vi "cDAQ_VI_Leo_Main.vi"() -> ()   [LabVIEW 2022 SP3]
uses:
  <vilib>/Analysis/baseanly.llb/Mean (DBL).vi
  <vilib>/DAQmx/read.llb/DAQmx Read (Analog 1D Wfm NChan NSamp).vi
  STOP_GLOBAL.vi
  <vilib>/addons/control/pid/pid.llb/PID Lead-Lag (DBL).vi
  <vilib>/addons/control/pid/pid.llb/PID (DBL).vi
  <vilib>/DAQmx/configure/timing.llb/DAQmx Timing (Sample Clock).vi
  <vilib>/DAQmx/miscellaneous.llb/DAQmx Fill In Error Info.vi
  <vilib>/Analysis/NI_AALBase.lvlib
  <vilib>/addons/control/pid/NI_PID_pid.lvlib
panel:
  out "Setpoint profile":dbl
  out "Voltage Output":dynamicdata(graph)
  out "Second Pressure Transducer":cluster{dbl[], dbl[]}(graph)
  out "Second Pressure Transducer":dynamicdata(graph)
  out "output":dbl format="%.2f"
  out "Servo Voltage Output":cluster{dbl[], dbl[]}(graph)
  out "Elapsed Time (s)":dbl
  in  "Tab Control":T1(tab)
  in  "Channel Array":dbl[](array[numeric]) format="%_3g"
  out "error out 5":errorcluster
  in  "stop":bool
  out "Output":dbl(slide) scale=0.0..5.067
  out "elapsed time (s)":dbl format="%.3f"
  in  "reinitialize? (F)":bool
  out "Waveform Chart 2":cluster{"setpoint":dbl, dbl}(graph) caption="Waveform Chart"
  out "Process Variable vs Setpoint":cluster{dbl[], dbl[]}[](graph)
  out "error out":errorcluster
  out "Steps on Needle 3":dbl[](array[numeric])
  in  "Error":dbl
  in  "Scaling Factor":dbl
  in  "x0":dbl
  out "element":dbl
  out "Process variable":dbl
  out "Setpoint":dbl
  in  "setpoint profile":cluster{"time (s)":dbl, "setpoint":dbl}[](array[cluster]) {"setpoint" format="%.2f"; "time (s)" format="%.3f"}
  in  "PID gains":T2={"proportional gain (Kc)"=1.0, "integral time (Ti, min)"=0.01, "derivative time (Td, min)"=0.0} {"derivative time (Td, min)" format="%.3f"; "integral time (Ti, min)" format="%.3f"; "proportional gain (Kc)" format="%.3f"}
  out "Steps on Servo":dbl[](array[numeric])
  out "Elapsed Time (s) 2":dbl caption="Elapsed Time (s)"
  out "HAS 3 SECONDS PASSED?":bool
  in  "PRESS TO START":bool
  out "All Channel Graph":cluster{dbl[], dbl[]}[](graph)
  out "Thrust":cluster{dbl[], dbl[]}(graph)
  out "Chamber Pressure":cluster{dbl[], dbl[]}(graph)
  out "Supply Pressure":cluster{dbl[], dbl[]}(graph)
  out "MassFlow":cluster{dbl[], dbl[]}(graph)
  out "Temperature":cluster{dbl[], dbl[]}(graph)
  out "error out 3":errorcluster caption="error out"
  out "error out 2":errorcluster
  in  "rate":dbl=1000.0 format="%0.2f"
  in  "number of samples":i32=100
  in  "File Format":string
  in  "File Name Out":string
  in  "Data Collection Folder":path
  out "Temperature":dynamicdata(graph)
  out "Numeric 2":i32
  out "Thrust lb":dynamicdata(graph)
  in  "Types of Testing":enum32{"Test Firing", "Cold Flow Rig"}(tab)
  out "Saving Data":bool
  out "Filename Out":path
  in  "Collect Data?":bool=TRUE caption="Enable"
  in  "Collect Data? 2":bool=TRUE caption="Enable"
  out "Saving Data":bool
  out "Filename Out":path
  out "Supply Pressure PSI":dynamicdata(graph)
  out "Mass Flow L/min":dynamicdata(graph)
  out "Chamber Pressure":dynamicdata(graph)
  # "Control Loop"
  # "DATA LOGGING INFORMATION"
  # "ANALOG VOLTAGE OUTPUT"
  # "RESULTS"
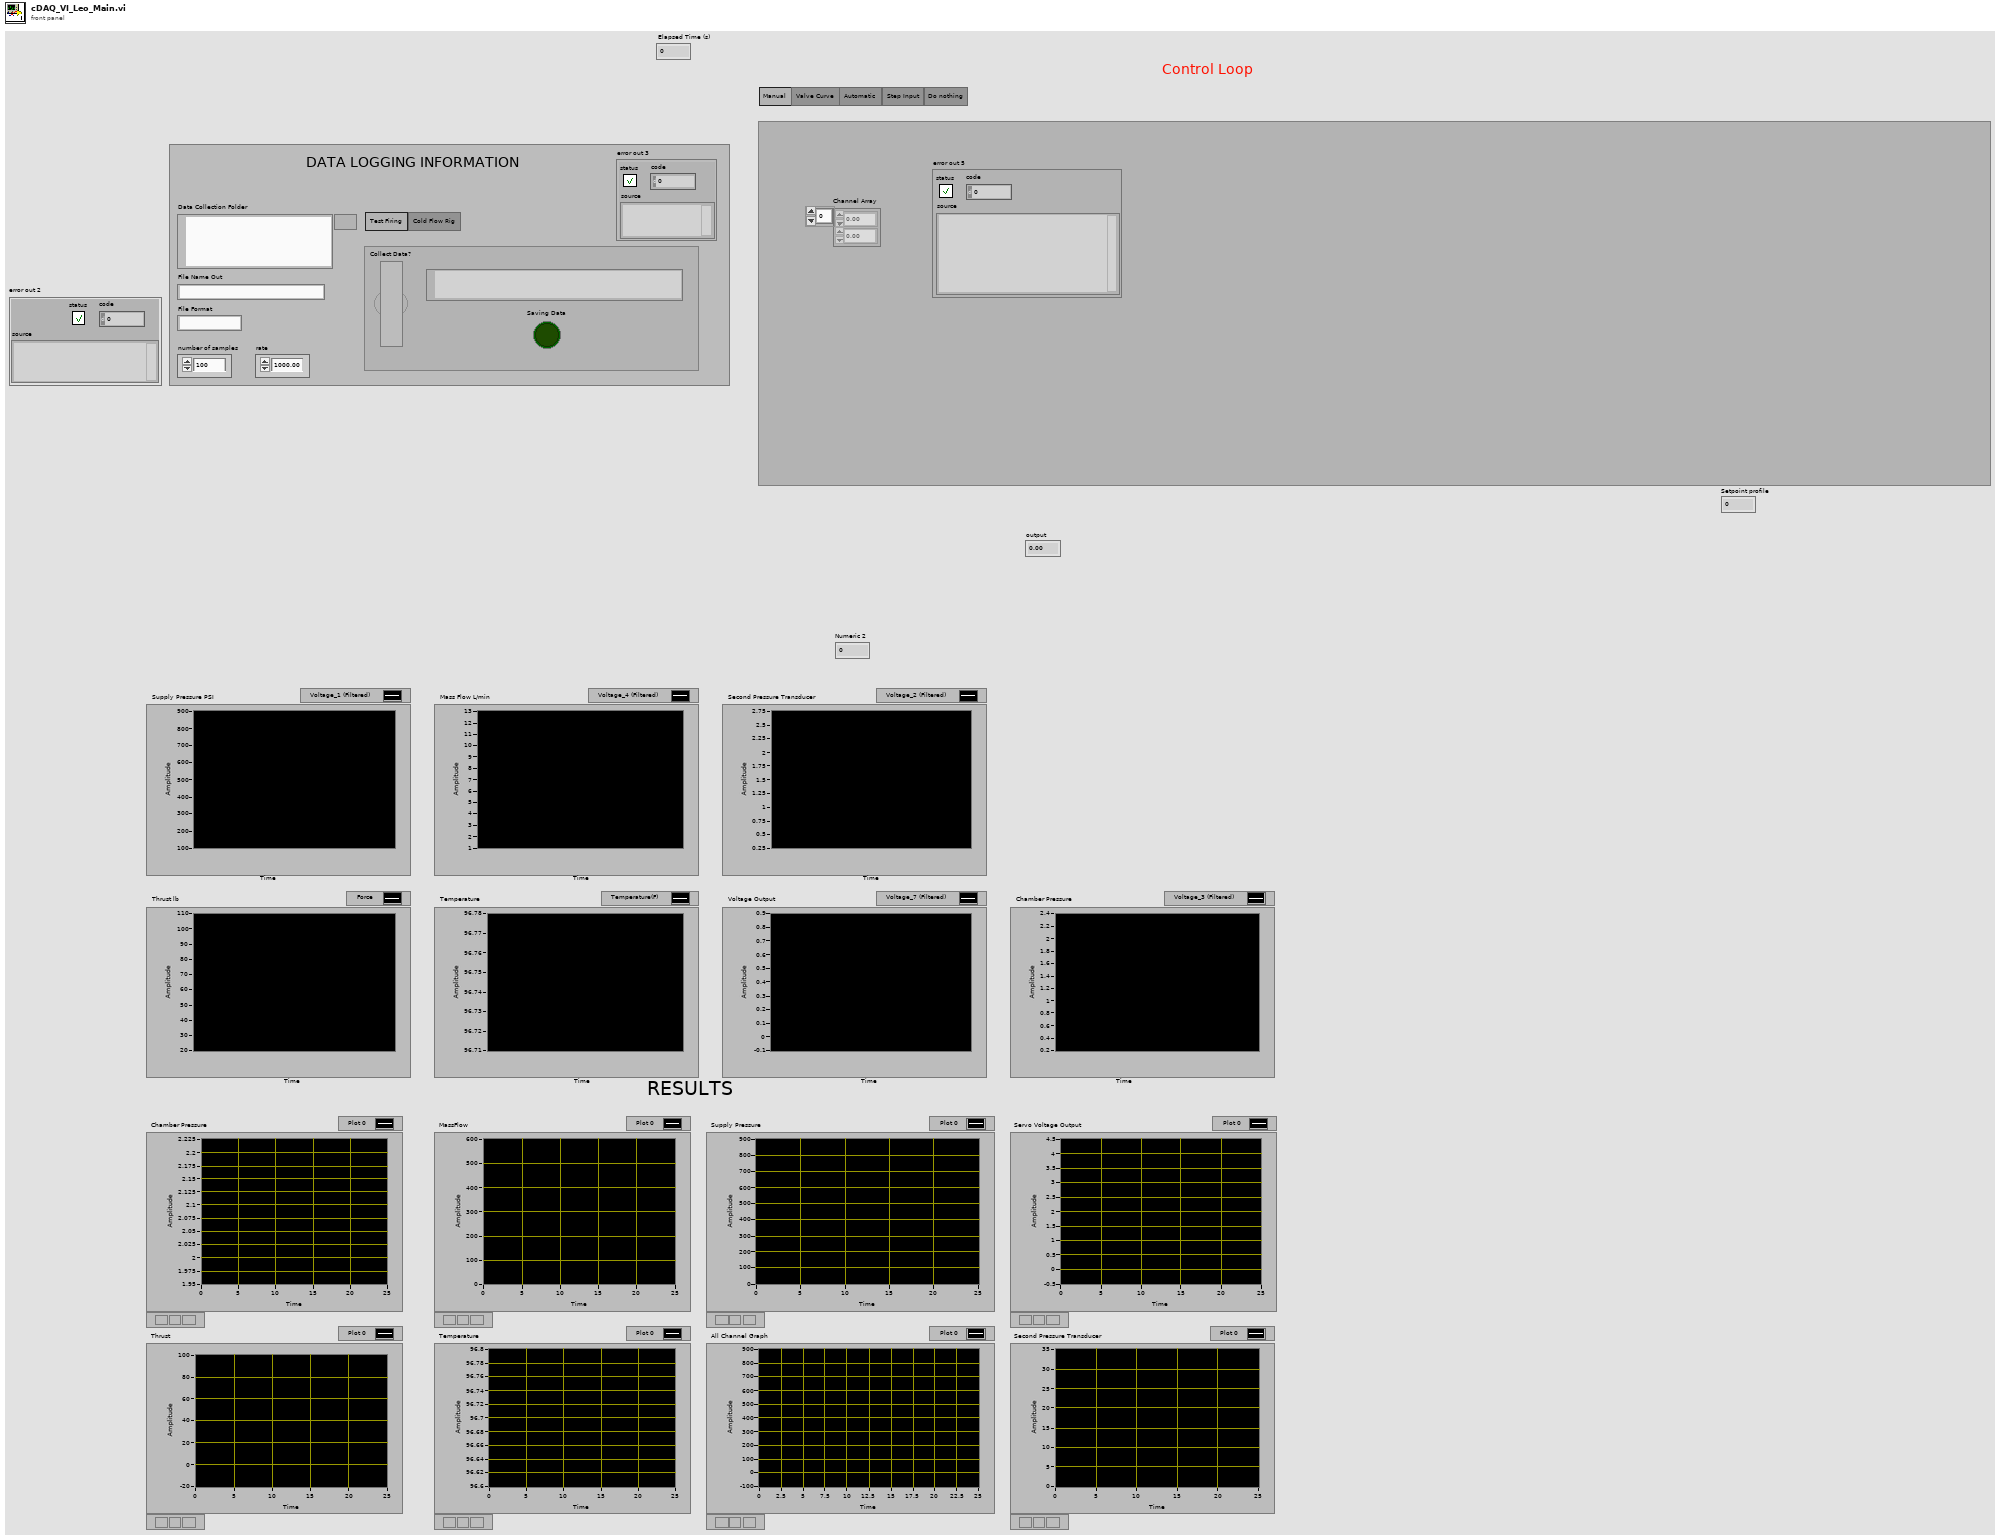
[diagram p1: front panel]
types:
  T1 = enum32{"Manual", "Valve Curve", "Automatic", "Step Input", "Do nothing"}
  T2 = cluster{"proportional gain (Kc)":dbl, "integral time (Ti, min)":dbl, "derivative time (Td, min)":dbl}
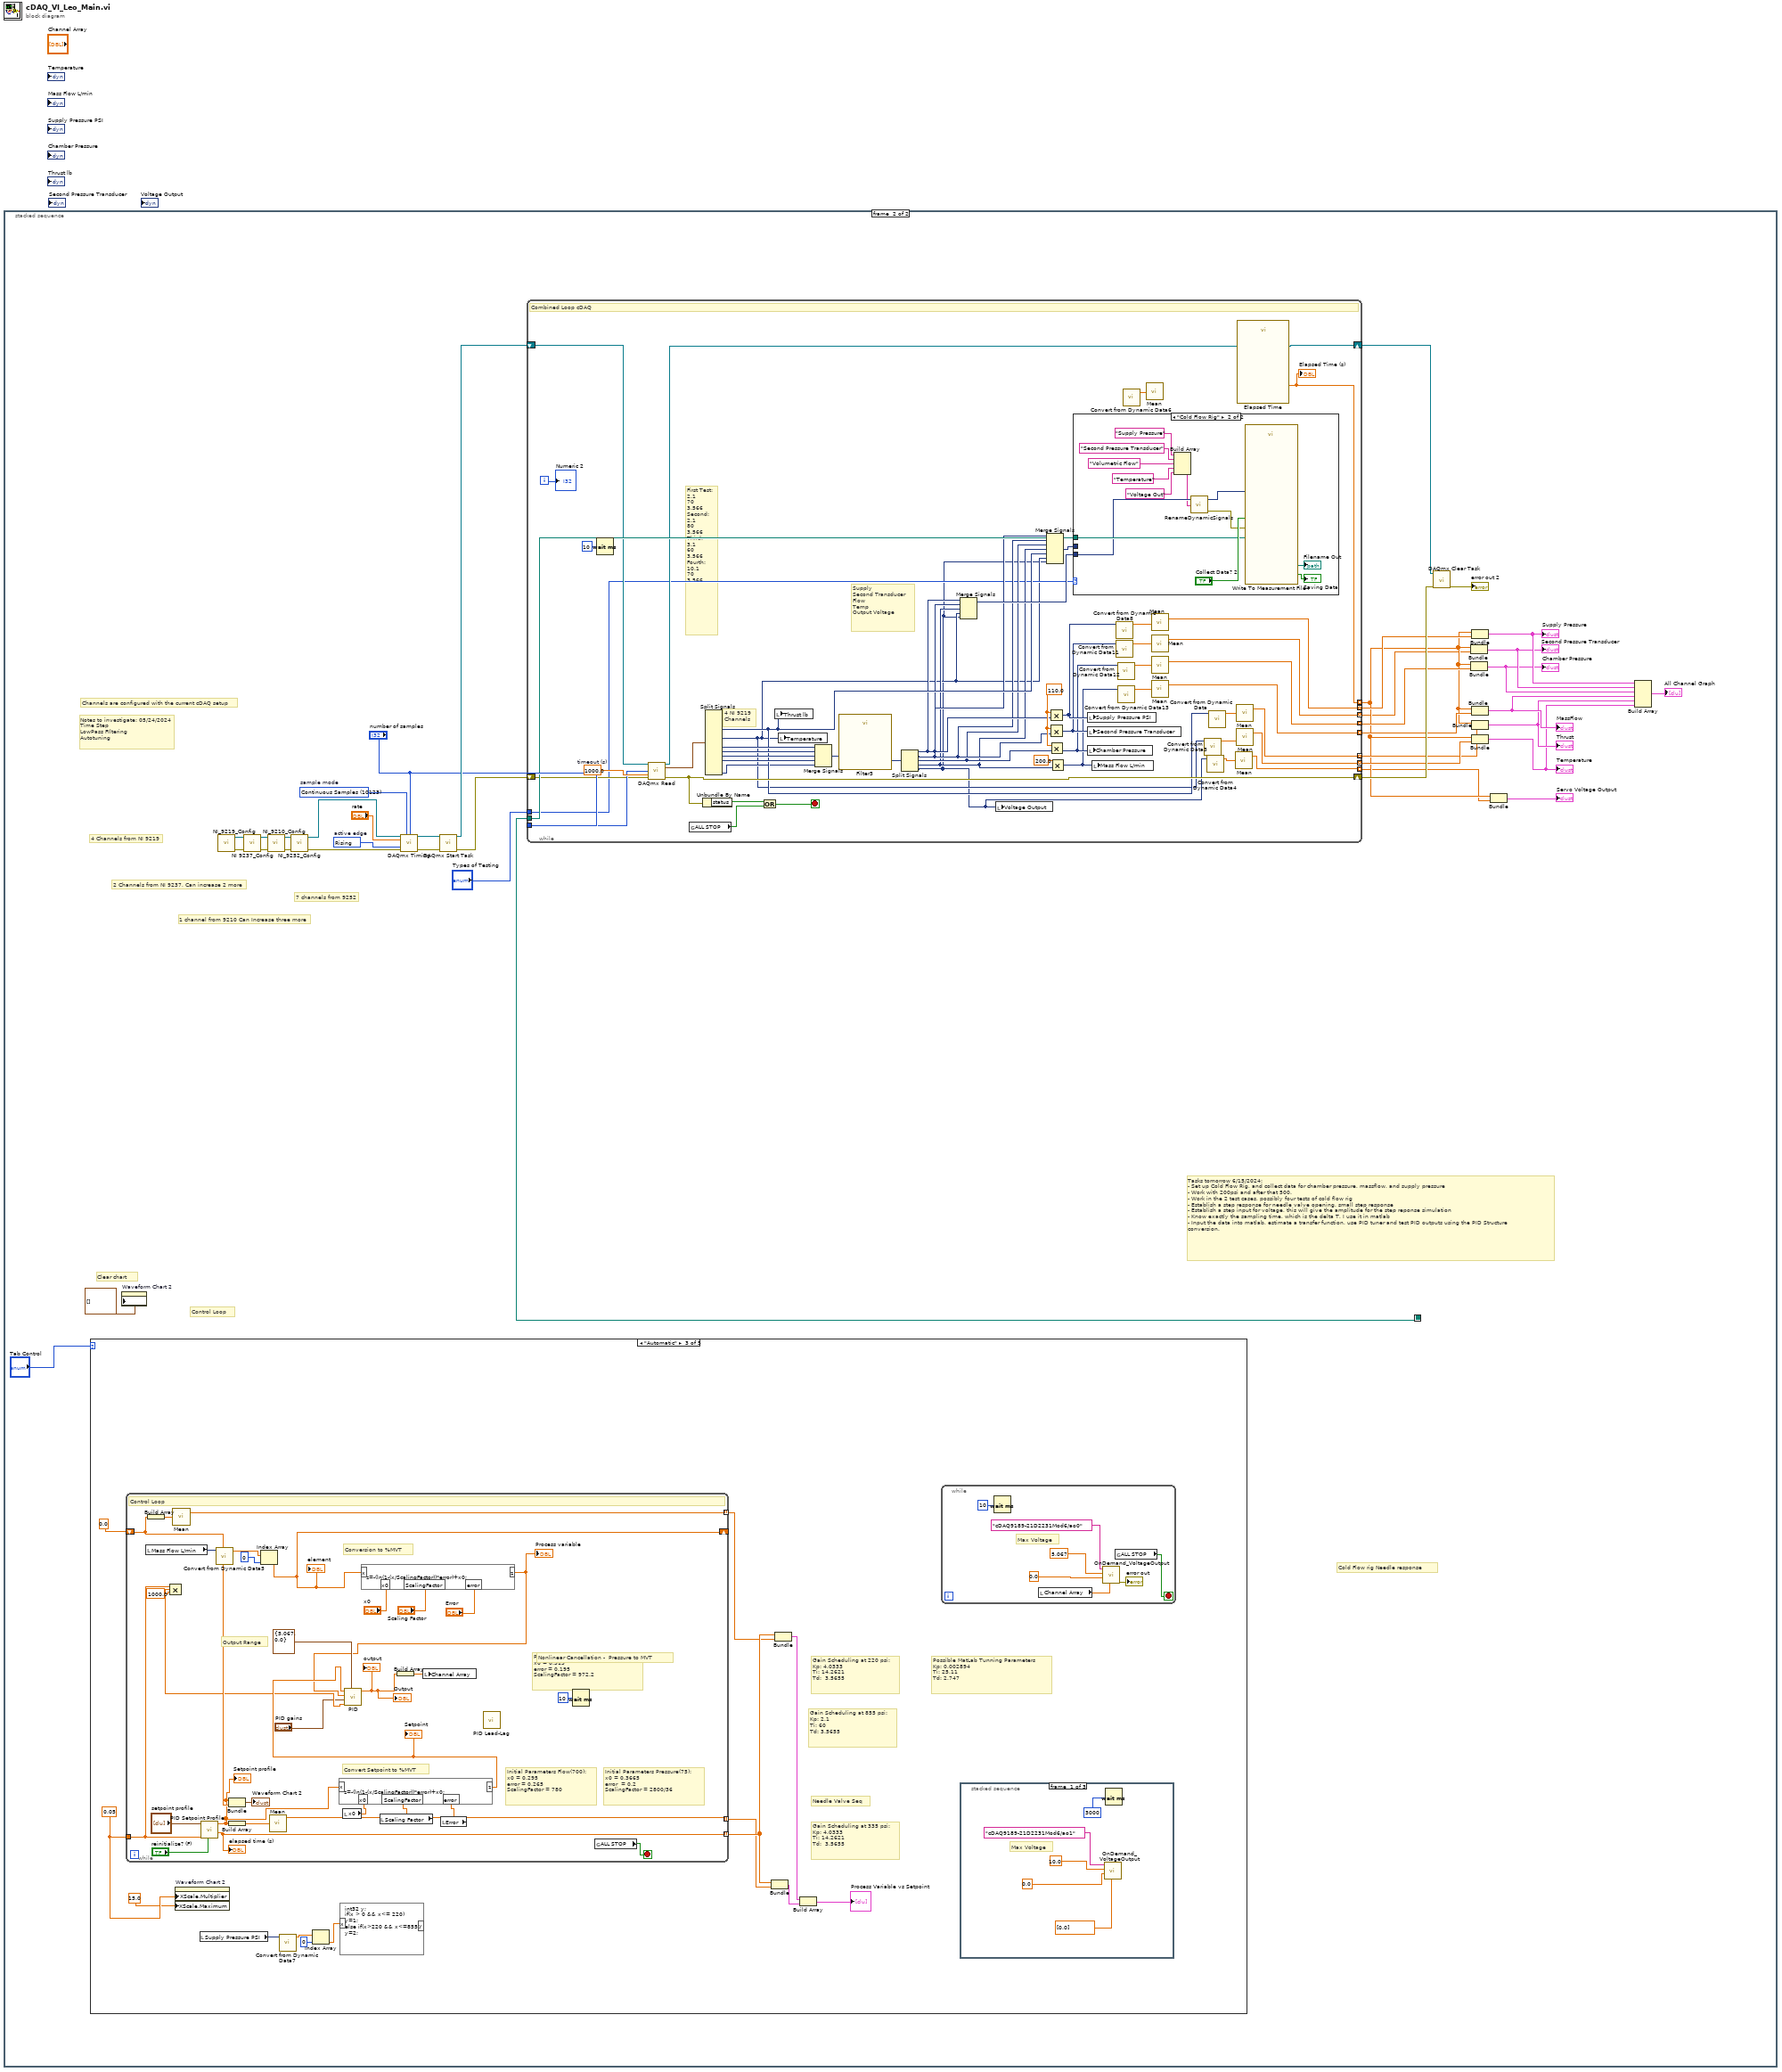
[diagram p0: block diagram]
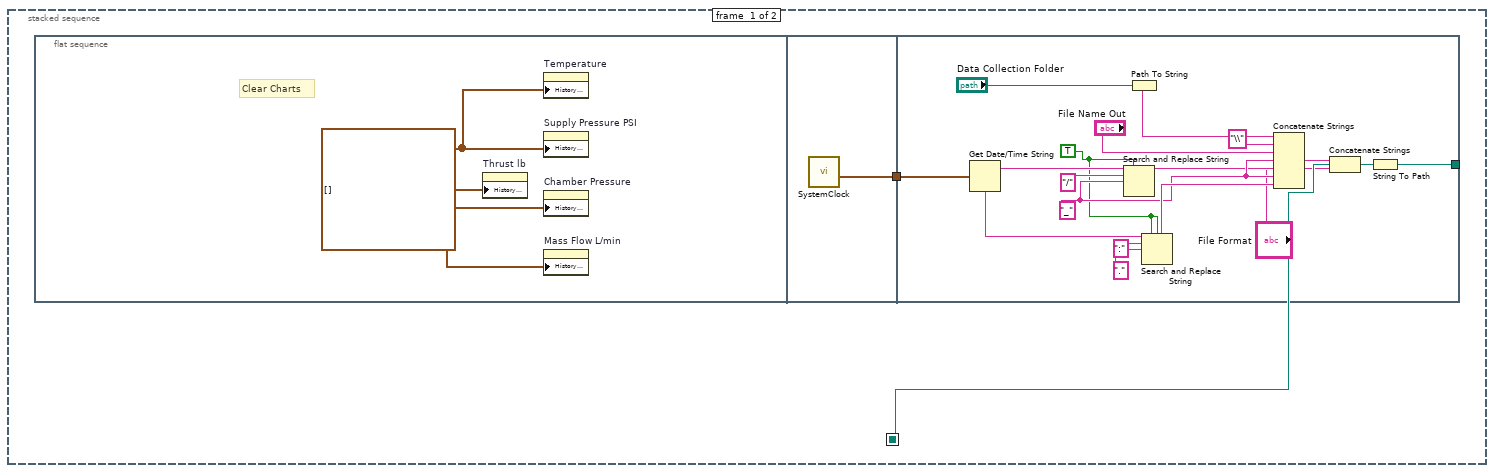
[diagram p2: hidden frame]
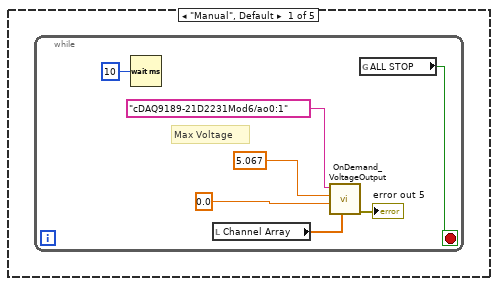
[diagram p3: hidden frame]
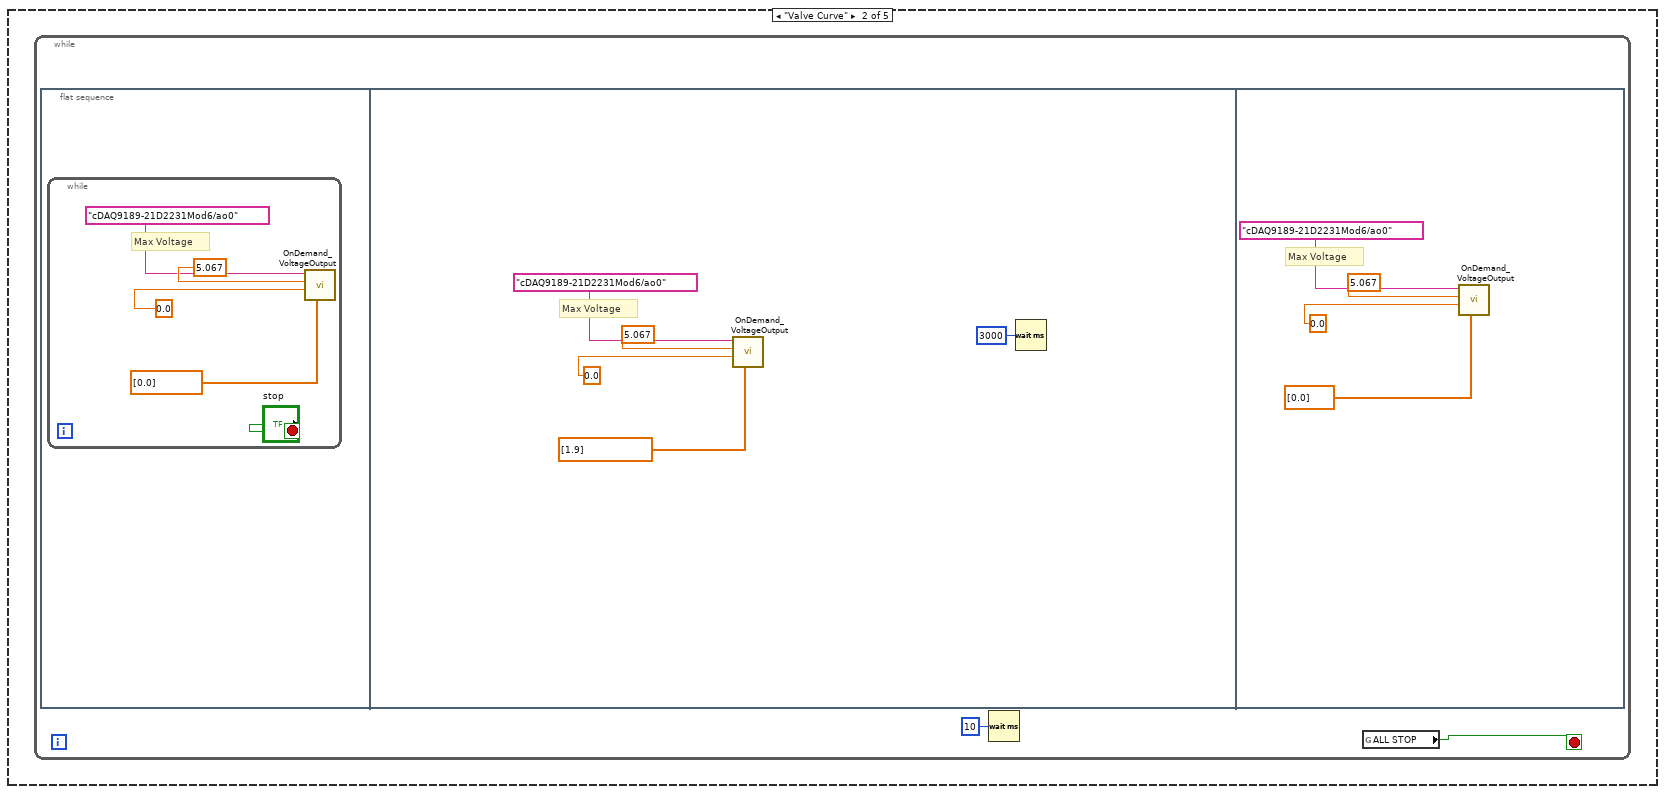
[diagram p4: hidden frame]
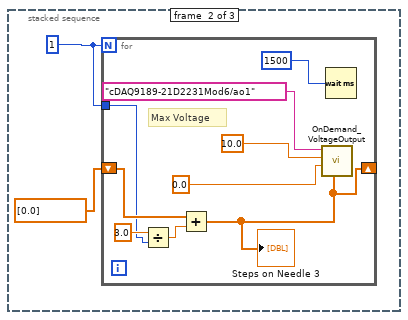
[diagram p5: hidden frame]
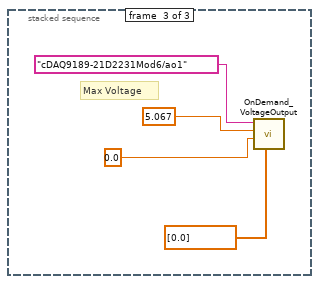
[diagram p6: hidden frame]
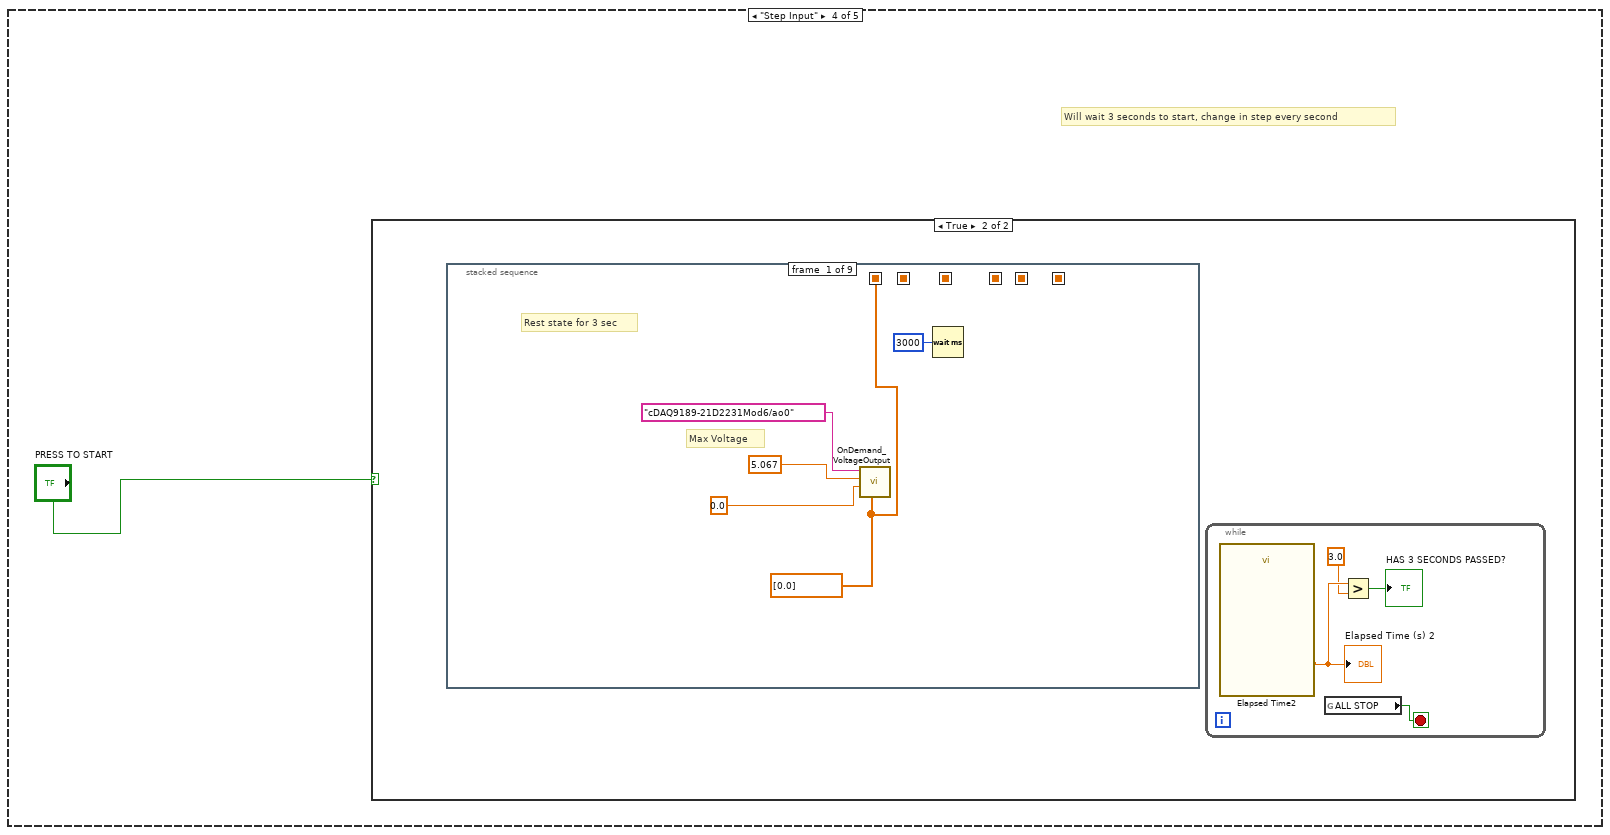
[diagram p7: hidden frame]
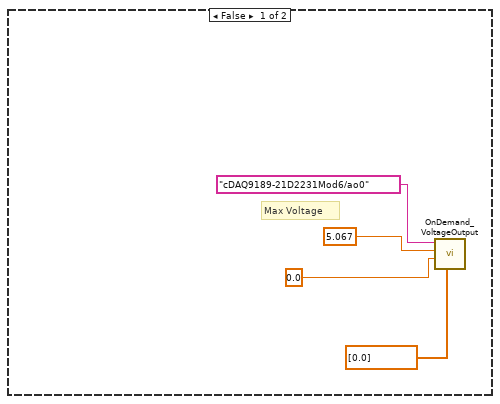
[diagram p8: hidden frame]
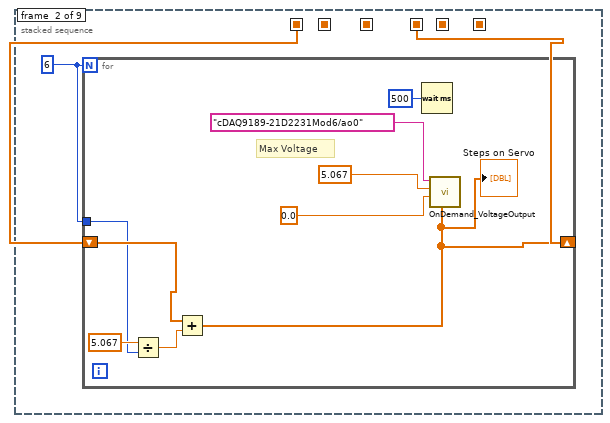
[diagram p9: hidden frame]
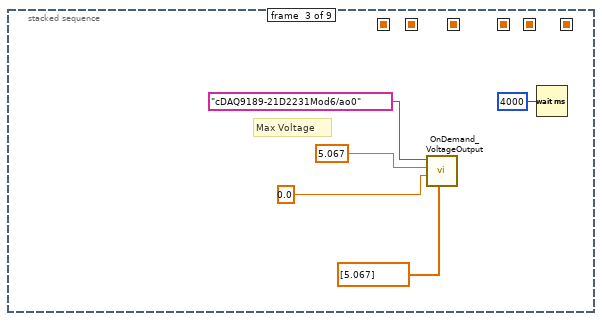
[diagram p10: hidden frame]
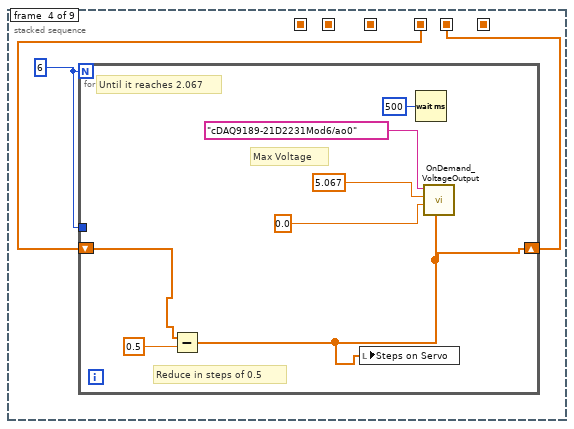
[diagram p11: hidden frame]
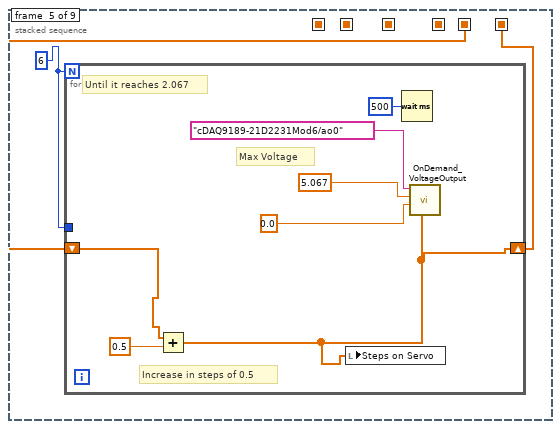
[diagram p12: hidden frame]
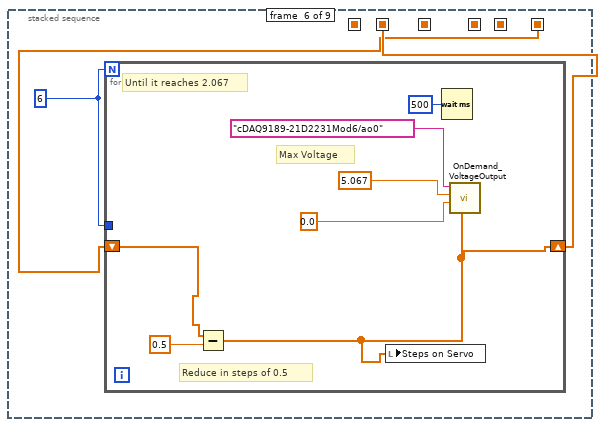
[diagram p13: hidden frame]
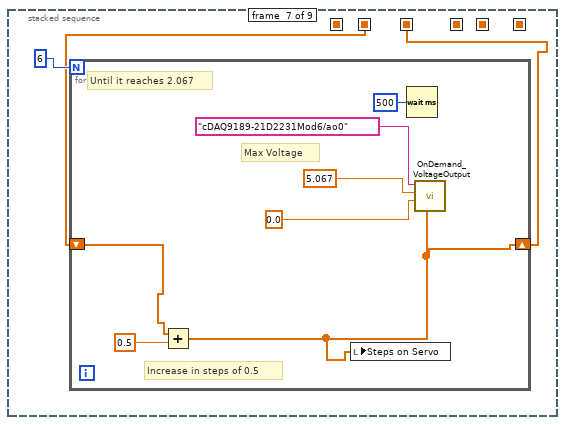
[diagram p14: hidden frame]
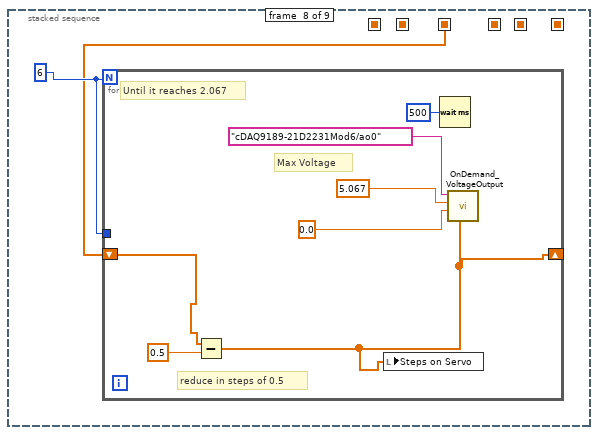
[diagram p15: hidden frame]
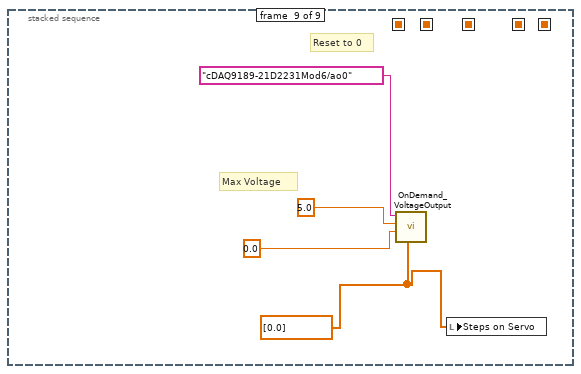
[diagram p16: hidden frame]
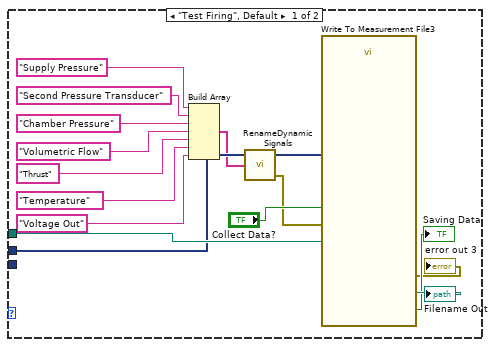
[diagram p18: hidden frame]
diagram:
  n1 = stacked-sequence {
    seq-local: [w1 _] -> [_ w60]
    frame #0 {
      n2 = flat-sequence {
        tunnel: [w4] -> w2
        tunnel: w2 -> [w11]
        tunnel: [w10] -> w1
        frame #0 {
          w3 = waveform(dbl)[] []
          # "Clear Charts"
          n3 = property on="Thrust lb" class="WFChart (strict)"("History Data"=w3) -> ()  [unwired: 2 in, 2 out]
          n4 = property on="Temperature" class="WFChart (strict)"("History Data"=w3) -> ()  [unwired: 2 in, 2 out]
          n5 = property on="Supply Pressure PSI" class="WFChart (strict)"("History Data"=w3) -> ()  [unwired: 2 in, 2 out]
          n6 = property on="Chamber Pressure" class="WFChart (strict)"("History Data"=w3) -> ()  [unwired: 2 in, 2 out]
          n7 = property on="Mass Flow L/min" class="WFChart (strict)"("History Data"=w3) -> ()  [unwired: 2 in, 2 out]
        }
        frame #1 {
          n8 = call "SystemClock.vi"() -> ("LabVIEW Time Stamp"=w4:timestamp)  [unwired: 9 in, 2 out]
        }
        frame #2 {
          w6 = TRUE ("replace all? (F)")
          w19 = "_" ("string")
          n9 = Get Date/Time String(seconds (now)=w11) -> (date string=w13:string, time string=w16:string)  [unwired: 2 in]
          n10 = Search and Replace String(replace all?=w6, input string=w13, search string="/", replace string=w19) -> (result string=w15:string)  [unwired: 4 in, 3 out]
          n11 = Path To String(path="Data Collection Folder") -> (string=w8:string)
          n12 = Search and Replace String(replace all?=w6, case sensitive?=w6, input string=w16, search string=":", replace string="." ("replace string (\"\")")) -> (result string=w20:string)  [unwired: 3 in, 3 out]
          n13 = Concatenate Strings(w8, "\\" ("string"), "File Name Out", w19, w15, w19, w20) -> (w21:string)
          n14 = Concatenate Strings(w21, "File Format") -> (w22:string)
          n15 = String To Path(string=w22) -> (path=w10:path)
        }
      }
    }
    frame #1 {
      w58 = 10123 items=["Finite Samples"=10178, "Continuous Samples"=10123, "Hardware Timed Single Point"=12522]  # sample mode
      w59 = 10280 items=["Rising"=10280, "Falling"=10171]  # active edge
      # "Cold Flow rig Needle response"
      # "Tasks tomorrow 6/15/2024:\n- Set up Cold Flow Rig, and collect data for chamber pressure, massflow, and supply pressure\n- Work with 200psi and after that 500.\n- Work in the 2 test cases, possibly four tests of cold flow rig\n- Establish a step response for needle valve opening, small step response\n- Establish a step input for voltage, this will give the amplitude for the step reponse simulation\n- Know exactly the sampling time, which is the delta T, I use it in matlab\n- Input the data into matlab, estimate a transfer function, use PID tuner and test PID outputs using the PID Structure\nconversion."
      # "Control Loop"
      # "Clear chart"
      # "Notes to investigate: 05/24/2024\nTime Step\nLowPass FIltering\nAutotuning"
      # "Channels are configured with the current cDAQ setup"
      # "7 channels from 9252"
      # "1 channel from 9210 Can Increase three more"
      # "2 Channels from NI 9237, Can increase 2 more"
      # "4 Channels from NI 9219"
      n16 = case shown="\"Automatic\"" "Tab Control" {
        frame "Manual", Default {
          n17 = while {
            stop <- w68 stop-if-true
            # "Max Voltage"
            n18 = Wait (ms)(milliseconds to wait=u32 10) -> ()  [unwired: 1 out]
            n19 = local read "Channel Array"() -> (w64:dbl[])
            n20 = call "OnDemand_VoltageOutput.vi"("Channel Array"=w64, "minimum voltage"=0.0, "maximum voltage"=5.067, "physical channels"="cDAQ9189-21D2231Mod6/ao0:1") -> ("error out"=→"error out 5":errorcluster)  [unwired: 7 in]
            n21 = global read "STOP_GLOBAL.vi" "ALL STOP"() -> (w68:bool)
          }
        }
        frame "Valve Curve" {
          n22 = while {
            stop <- w69 stop-if-true
            n23 = flat-sequence {
              frame #0 {
                n24 = while {
                  stop <- "stop" stop-if-true
                  # "Max Voltage"
                  n25 = call "OnDemand_VoltageOutput.vi"("Channel Array"=dbl[] [0.0], "minimum voltage"=0.0, "maximum voltage"=5.067, "physical channels"="cDAQ9189-21D2231Mod6/ao0") -> ()  [unwired: 7 in, 1 out]
                }
              }
              frame #1 {
                # "Max Voltage"
                n26 = call "OnDemand_VoltageOutput.vi"("Channel Array"=dbl[] [1.9], "minimum voltage"=0.0, "maximum voltage"=5.067, "physical channels"="cDAQ9189-21D2231Mod6/ao0") -> ()  [unwired: 7 in, 1 out]
                n27 = Wait (ms)(milliseconds to wait=u32 3000) -> ()  [unwired: 1 out]
              }
              frame #2 {
                # "Max Voltage"
                n28 = call "OnDemand_VoltageOutput.vi"("Channel Array"=dbl[] [0.0], "minimum voltage"=0.0, "maximum voltage"=5.067, "physical channels"="cDAQ9189-21D2231Mod6/ao0") -> ()  [unwired: 7 in, 1 out]
              }
            }
            n29 = Wait (ms)(milliseconds to wait=u32 10) -> ()  [unwired: 1 out]
            n30 = global read "STOP_GLOBAL.vi" "ALL STOP"() -> (w69:bool)
          }
        }
        frame "Automatic" {
          w97 = 0.05 ("dt (s)")
          # "Possible MatLab Tunning Parameters\nKp: 0.002894\nTi: 25.11\nTd: 2.747"
          # "Gain Scheduling at 335 psi:\nKp: 4.0333\nTi: 14.2621\nTd:  3.5655"
          # "Gain Scheduling at 855 psi:\nKp: 2.1\nTi: 60\nTd: 3.5655"
          # "Gain Scheduling at 220 psi:\nKp: 4.0333\nTi: 14.2621\nTd:  3.5655"
          # "Needle Valve Seq"
          n31 = while {
            shift-right: [w132] -> _
            shift-left: 0.0 -> [w149]
            tunnel: w97 -> [w152]
            tunnel: [w150] -> w93 mode=indexing
            tunnel: [w148] -> w91 mode=indexing
            tunnel: [w146] -> w92 mode=indexing
            stop <- w155 stop-if-true
            # "Possible parameters for 800 SLM:\nx0 = 0.315\nerror = 0.195\nScalingFactor = 972.2"
            # "Initial Parameters Pressure(75):\nx0 = 0.3665\nerror  = 0.2\nScalingFactor = 2800/36"
            # "Initial Parameters Flow(700):\nx0 = 0.295\nerror = 0.265\nScalingFactor = 780"
            # "Nonlinear Cancellation -  Pressure to MVT"
            # "Convert Setpoint to %MVT"
            # "Conversion to %MVT"
            # "Output Range"
            # "Control Loop"
            n32 = local read "Mass Flow L/min"() -> (w128:dynamicdata)
            n33 = Build Array(w149) -> (w147:dbl[])
            n34 = Multiply(x=w152, y=1000.0) -> (x*y=w136:dbl)
            n35 = call-poly <vilib>:"Mean.vi"("X"=w147) -> ("mean"=w148:dbl)  [unwired: 1 out]
            n36 = call <vilib>:"PID Setpoint Profile.vi"("reinitialize? (F)"="reinitialize? (F)", "dt (s)"=w152, "setpoint profile"="setpoint profile") -> ("elapsed time (s)"=w150:dbl, "setpoint"=w126:dbl)  [unwired: 3 in, 2 out]
            "elapsed time (s)" <- w150
            "Setpoint profile" <- w126
            n37 = call "Convert from Dynamic Data5"("Dynamic Data Type"=w128) -> ("Array"=w131:dbl[])  [unwired: 3 in]
            n38 = Bundle("setpoint"=w126, w149) -> (→"Waveform Chart 2":cluster{"setpoint":dbl, dbl})  [unwired: 1 in]
            n39 = Build Array(w126) -> (w143:dbl[])
            n40 = Index Array(array=w131, index=0) -> (element=w132:dbl)
            "element" <- w132
            n41 = call-poly <vilib>:"Mean.vi"("X"=w143) -> ("mean"=w146:dbl)  [unwired: 1 out]
            n42 = local read "x0"() -> (w142:dbl)
            n43 = formula code="z=-(ln(1-(x/ScalingFactor))*error)+x0;"("x"=w132, "x0"="x0", "ScalingFactor"="Scaling Factor", "error"="Error") -> ("z"=w129:dbl)
            "Process variable" <- w129
            n44 = local read "Scaling Factor"() -> (w141:dbl)
            n45 = local read "Error"() -> (w140:dbl)
            n46 = formula code="z=-(ln(1-(x/ScalingFactor))*error)+x0;"("x"=w126, "x0"=w142, "ScalingFactor"=w141, "error"=w140) -> ("z"=w137:dbl)
            "Setpoint" <- w137
            n47 = call-poly <vilib>:"PID.vi"("output range"=cluster{"output high":dbl, "output low":dbl} {"output high"=5.067, "output low"=0.0}, "dt (s)"=w136, "PID gains"="PID gains", "process variable"=w129, "setpoint"=w137) -> ("output"=w139:dbl)  [unwired: 5 in, 1 out]
            "Output" <- w139
            "output" <- w139
            n48 = Build Array(w139) -> (w151:dbl[])
            n49 = local write "Channel Array"(w151) -> ()
            n50 = call-poly <vilib>:"PID Lead-Lag.vi"() -> ()  [unwired: 8 in, 2 out]
            n51 = Wait (ms)(milliseconds to wait=u32 10) -> ()  [unwired: 1 out]
            n52 = global read "STOP_GLOBAL.vi" "ALL STOP"() -> (w155:bool)
          }
          n53 = property on="Waveform Chart 2" class="WFChart (strict)"("XScale.Multiplier"=w97, "XScale.Maximum"=15.0 ("X Scale.Range:Maximum")) -> ()  [unwired: 2 in, 2 out]
          n54 = local read "Supply Pressure PSI"() -> (w88:dynamicdata)
          n55 = call "Convert from Dynamic Data7"("Dynamic Data Type"=w88) -> ("Array"=w87:dbl[])  [unwired: 3 in]
          n56 = Index Array(array=w87, index=0) -> (element=w85:dbl)
          n57 = formula code="int32 y;\nif(x > 0 && x<= 220)\ny=1;\nelse if(x>220 && x<=855)\ny=2;"("x"=w85) -> ()  [unwired: 1 out]
          n58 = Bundle(w93, w92) -> (w94:cluster{dbl[], dbl[]})  [unwired: 1 in]
          n59 = Bundle(w93, w91) -> (w89:cluster{dbl[], dbl[]})  [unwired: 1 in]
          n60 = Build Array(w89, w94) -> (→"Process Variable vs Setpoint":cluster{dbl[], dbl[]}[])
          n61 = while {
            stop <- w124 stop-if-true
            # "Max Voltage"
            n62 = Wait (ms)(milliseconds to wait=u32 10) -> ()  [unwired: 1 out]
            n63 = local read "Channel Array"() -> (w120:dbl[])
            n64 = call "OnDemand_VoltageOutput.vi"("Channel Array"=w120, "minimum voltage"=0.0, "maximum voltage"=5.067, "physical channels"="cDAQ9189-21D2231Mod6/ao0") -> ("error out"=→"error out":errorcluster)  [unwired: 7 in]
            n65 = global read "STOP_GLOBAL.vi" "ALL STOP"() -> (w124:bool)
          }
          n66 = stacked-sequence {
            frame #0 {
              # "Max Voltage"
              n67 = call "OnDemand_VoltageOutput.vi"("Channel Array"=dbl[] [0.0], "minimum voltage"=0.0, "maximum voltage"=10.0, "physical channels"="cDAQ9189-21D2231Mod6/ao1") -> ()  [unwired: 7 in, 1 out]
              n68 = Wait (ms)(milliseconds to wait=u32 3000) -> ()  [unwired: 1 out]
            }
            frame #1 {
              w103 = 1
              n69 = for {
                N: w103 -> [_]
                shift-right: [w105] -> _
                shift-left: dbl[] [0.0] -> [w109]
                tunnel: w103 -> [w107]
                # "Max Voltage"
                n70 = Divide(x=3.0, y=w107) -> (x/y=w106:dbl)
                n71 = Add(x=w109, y=w106) -> (x+y=w105:dbl[])
                "Steps on Needle 3" <- w105
                n72 = call "OnDemand_VoltageOutput.vi"("Channel Array"=w105, "minimum voltage"=0.0, "maximum voltage"=10.0, "physical channels"="cDAQ9189-21D2231Mod6/ao1") -> ()  [unwired: 7 in, 1 out]
                n73 = Wait (ms)(milliseconds to wait=u32 1500) -> ()  [unwired: 1 out]
              }
            }
            frame #2 {
              # "Max Voltage"
              n74 = call "OnDemand_VoltageOutput.vi"("Channel Array"=dbl[] [0.0], "minimum voltage"=0.0, "maximum voltage"=5.067, "physical channels"="cDAQ9189-21D2231Mod6/ao1") -> ()  [unwired: 7 in, 1 out]
            }
          }
        }
        frame "Step Input" {
          # "Will wait 3 seconds to start, change in step every second"
          n75 = case shown="True" "PRESS TO START" {
            frame False {
              # "Max Voltage"
              n76 = call "OnDemand_VoltageOutput.vi"("Channel Array"=dbl[] [0.0], "minimum voltage"=0.0, "maximum voltage"=5.067, "physical channels"="cDAQ9189-21D2231Mod6/ao0") -> ()  [unwired: 7 in, 1 out]
            }
            frame True {
              n77 = stacked-sequence {
                seq-local: [_ _ _ _ _ w208 _ _ _] -> [_ _ _ _ _ _ w218 _ _]
                seq-local: [_ _ _ _ _ _ w217 _ _] -> [_ _ _ _ _ _ _ w227 _]
                seq-local: [w165 _ _ _ _ _ _ _ _] -> [_ w171 _ _ _ _ _ _ _]
                seq-local: [_ w170 _ _ _ _ _ _ _] -> [_ _ _ w188 _ _ _ _ _]
                seq-local: [_ _ _ w187 _ _ _ _ _] -> [_ _ _ _ w198 _ _ _ _]
                seq-local: [_ _ _ _ w197 _ _ _ _] -> [_ _ _ _ _ w207 _ _ _]
                frame #0 {
                  w165 = dbl[] [0.0]
                  # "Rest state for 3 sec"
                  # "Max Voltage"
                  n78 = call "OnDemand_VoltageOutput.vi"("Channel Array"=w165, "minimum voltage"=0.0, "maximum voltage"=5.067, "physical channels"="cDAQ9189-21D2231Mod6/ao0") -> ()  [unwired: 7 in, 1 out]
                  n79 = Wait (ms)(milliseconds to wait=u32 3000) -> ()  [unwired: 1 out]
                }
                frame #1 {
                  w172 = 6
                  n80 = for {
                    N: w172 -> [_]
                    shift-right: [w173] -> w170
                    shift-left: w171 -> [w180]
                    tunnel: w172 -> [w174]
                    # "Max Voltage"
                    n81 = Divide(x=5.067, y=w174) -> (x/y=w176:dbl)
                    n82 = Add(x=w180, y=w176) -> (x+y=w173:dbl[])
                    "Steps on Servo" <- w173
                    n83 = Wait (ms)(milliseconds to wait=u32 500) -> ()  [unwired: 1 out]
                    n84 = call "OnDemand_VoltageOutput.vi"("Channel Array"=w173, "minimum voltage"=0.0, "maximum voltage"=5.067, "physical channels"="cDAQ9189-21D2231Mod6/ao0") -> ()  [unwired: 7 in, 1 out]
                  }
                }
                frame #2 {
                  # "Max Voltage"
                  n85 = call "OnDemand_VoltageOutput.vi"("Channel Array"=dbl[] [5.067], "minimum voltage"=0.0, "maximum voltage"=5.067, "physical channels"="cDAQ9189-21D2231Mod6/ao0") -> ()  [unwired: 7 in, 1 out]
                  n86 = Wait (ms)(milliseconds to wait=u32 4000) -> ()  [unwired: 1 out]
                }
                frame #3 {
                  w189 = 6
                  n87 = for {
                    N: w189 -> [_]
                    shift-right: [w190] -> w187
                    shift-left: w188 -> [w196]
                    tunnel: w189 -> [_]
                    # "Max Voltage"
                    # "Until it reaches 2.067"
                    # "Reduce in steps of 0.5"
                    n88 = Subtract(x=w196, y=0.5) -> (x-y=w190:dbl[])
                    n89 = local write "Steps on Servo"(w190) -> ()
                    n90 = Wait (ms)(milliseconds to wait=u32 500) -> ()  [unwired: 1 out]
                    n91 = call "OnDemand_VoltageOutput.vi"("Channel Array"=w190, "minimum voltage"=0.0, "maximum voltage"=5.067, "physical channels"="cDAQ9189-21D2231Mod6/ao0") -> ()  [unwired: 7 in, 1 out]
                  }
                }
                frame #4 {
                  w199 = 6
                  n92 = for {
                    N: w199 -> [_]
                    shift-right: [w200] -> w197
                    shift-left: w198 -> [w206]
                    tunnel: w199 -> [_]
                    # "Max Voltage"
                    # "Until it reaches 2.067"
                    # "Increase in steps of 0.5"
                    n93 = Add(x=w206, y=0.5) -> (x+y=w200:dbl[])
                    n94 = local write "Steps on Servo"(w200) -> ()
                    n95 = Wait (ms)(milliseconds to wait=u32 500) -> ()  [unwired: 1 out]
                    n96 = call "OnDemand_VoltageOutput.vi"("Channel Array"=w200, "minimum voltage"=0.0, "maximum voltage"=5.067, "physical channels"="cDAQ9189-21D2231Mod6/ao0") -> ()  [unwired: 7 in, 1 out]
                  }
                }
                frame #5 {
                  w209 = 6
                  n97 = for {
                    N: w209 -> [_]
                    shift-right: [w210] -> w208
                    shift-left: w207 -> [w216]
                    tunnel: w209 -> [_]
                    # "Max Voltage"
                    # "Until it reaches 2.067"
                    # "Reduce in steps of 0.5"
                    n98 = Subtract(x=w216, y=0.5) -> (x-y=w210:dbl[])
                    n99 = local write "Steps on Servo"(w210) -> ()
                    n100 = Wait (ms)(milliseconds to wait=u32 500) -> ()  [unwired: 1 out]
                    n101 = call "OnDemand_VoltageOutput.vi"("Channel Array"=w210, "minimum voltage"=0.0, "maximum voltage"=5.067, "physical channels"="cDAQ9189-21D2231Mod6/ao0") -> ()  [unwired: 7 in, 1 out]
                  }
                }
                frame #6 {
                  n102 = for {
                    N: 6 -> [_]
                    shift-right: [w220] -> w217
                    shift-left: w218 -> [w226]
                    # "Max Voltage"
                    # "Until it reaches 2.067"
                    # "Increase in steps of 0.5"
                    n103 = Add(x=w226, y=0.5) -> (x+y=w220:dbl[])
                    n104 = local write "Steps on Servo"(w220) -> ()
                    n105 = Wait (ms)(milliseconds to wait=u32 500) -> ()  [unwired: 1 out]
                    n106 = call "OnDemand_VoltageOutput.vi"("Channel Array"=w220, "minimum voltage"=0.0, "maximum voltage"=5.067, "physical channels"="cDAQ9189-21D2231Mod6/ao0") -> ()  [unwired: 7 in, 1 out]
                  }
                }
                frame #7 {
                  w228 = 6
                  n107 = for {
                    N: w228 -> [_]
                    shift-right: [w229] -> _
                    shift-left: w227 -> [w235]
                    tunnel: w228 -> [_]
                    # "Max Voltage"
                    # "Until it reaches 2.067"
                    # "reduce in steps of 0.5"
                    n108 = Subtract(x=w235, y=0.5) -> (x-y=w229:dbl[])
                    n109 = local write "Steps on Servo"(w229) -> ()
                    n110 = Wait (ms)(milliseconds to wait=u32 500) -> ()  [unwired: 1 out]
                    n111 = call "OnDemand_VoltageOutput.vi"("Channel Array"=w229, "minimum voltage"=0.0, "maximum voltage"=5.067, "physical channels"="cDAQ9189-21D2231Mod6/ao0") -> ()  [unwired: 7 in, 1 out]
                  }
                }
                frame #8 {
                  w236 = dbl[] [0.0]
                  # "Reset to 0"
                  # "Max Voltage"
                  n112 = call "OnDemand_VoltageOutput.vi"("Channel Array"=w236, "minimum voltage"=0.0, "maximum voltage"=5.0, "physical channels"="cDAQ9189-21D2231Mod6/ao0") -> ()  [unwired: 7 in, 1 out]
                  n113 = local write "Steps on Servo"(w236) -> ()
                }
              }
              n114 = while {
                stop <- w164 stop-if-true
                n115 = call "Elapsed Time2"() -> ("Elapsed Time (s)"=w162:dbl)  [unwired: 12 in, 7 out]
                "Elapsed Time (s) 2" <- w162
                n116 = global read "STOP_GLOBAL.vi" "ALL STOP"() -> (w164:bool)
                n117 = Greater?(x=w162, y=3.0 ("x")) -> (0:→"HAS 3 SECONDS PASSED?":bool)
              }
            }
          }
        }
        frame "Do nothing" {
        }
      }
      n118 = property on="Waveform Chart 2" class="WFChart (strict)"("History Data"=cluster{"setpoint":dbl, dbl}[] []) -> ()  [unwired: 2 in, 2 out]
      n119 = call "NI_9219_Config.vi"() -> ("error out"=w43:errorcluster, "task out"=w51:refnum<k21>)  [unwired: 10 in]
      n120 = call "NI 9237_Config.vi"("error in"=w43, "task in"=w51) -> ("error out"=w49:errorcluster, "task out"=w50:refnum<k21>)  [unwired: 8 in]
      n121 = call "NI_9210_Config.vi"("error in"=w49, "task in"=w50) -> ("error out"=w47:errorcluster, "task out"=w48:refnum<k21>)  [unwired: 8 in]
      n122 = call "NI_9252_Config.vi"("error in"=w47, "task in"=w48) -> ("error out"=w45:errorcluster, "task out"=w46:refnum<k21>)  [unwired: 8 in]
      n123 = call-poly <vilib>:"DAQmx Timing.vi"("task/channels in"=w46, "sample mode"=w58, "samples per channel"="number of samples", "rate"="rate", "active edge"=w59, "error in"=w45) -> ("task out"=w57:refnum<k21>, "error out"=w56:errorcluster)  [unwired: 8 in]
      n124 = call <vilib>:"DAQmx Start Task.vi"("task/channels in"=w57, "error in"=w56) -> ("task out"=w55:refnum<k21>, "error out"=w54:errorcluster)  [unwired: 12 in]
      n125 = while {
        tunnel: "Types of Testing" -> [w244]
        tunnel: [w290] -> w39 mode=indexing
        tunnel: w60 -> [w285]
        tunnel: "number of samples" -> [w283]
        shift-right: [w277] -> w52
        shift-left: w54 -> [w282]
        shift-right: [w249] -> w53
        shift-left: w55 -> [w281]
        tunnel: [w260] -> w40 mode=indexing
        tunnel: [w258] -> w33 mode=indexing
        tunnel: [w257] -> w41 mode=indexing
        tunnel: [w256] -> w42 mode=indexing
        tunnel: [w251] -> w24 mode=indexing
        tunnel: [w250] -> w32 mode=indexing
        tunnel: [w259] -> w31 mode=indexing
        i -> [w291]
        stop <- w286 stop-if-true
        w271 = 110.0 ("x")
        w288 = 1000.0  # timeout (s)
        # "First Test:\n2.1\n70\n3.566\nSecond:\n2.1\n80\n3.566\nThird:\n3.1\n60\n3.566\nFourth:\n10.1\n70\n3.566"
        # "Supply\nSecond Transducer\nFlow\nTemp\nOutput Voltage"
        # "4 NI 9219 Channels"
        # "Combined Loop cDAQ"
        n126 = Wait (ms)(milliseconds to wait=u32 10) -> ()  [unwired: 1 out]
        n127 = call-poly <vilib>:"DAQmx Read.vi"("task/channels in"=w281, "number of samples per channel"=w283, "timeout"=w288, "error in"=w282) -> ("task out"=w249:refnum<k21>, "data"=w284:waveform(dbl)[], "error out"=w277:errorcluster)  [unwired: 9 in]
        n128 = global read "STOP_GLOBAL.vi" "ALL STOP"() -> (w287:bool)
        n129 = Unbundle By Name(w277) -> ("status"=w289:bool)
        n130 = Split Signals(w284) -> (w255:dynamicdata, w242:dynamicdata, w276:dynamicdata, w275:dynamicdata, w274:dynamicdata, w273:dynamicdata, w243:dynamicdata)  [unwired: 15 in, 8 out]
        n131 = Or(x=w289, y=w287) -> (x .or. y?=w286:bool)
        n132 = local write "Thrust lb"(w255) -> ()
        n133 = local write "Temperature"(w242) -> ()
        n134 = Merge Signals(w276, w275, w274, w273, w243) -> (w272:dynamicdata)
        n135 = call "Filter3"("Signal"=w272) -> ("Filtered Signal"=w269:dynamicdata)  [unwired: 9 in, 1 out]
        n136 = Split Signals(w269) -> (w248:dynamicdata, w247:dynamicdata, w246:dynamicdata, w245:dynamicdata, w240:dynamicdata)  [unwired: 5 in]
        n137 = Merge Signals(w248, w247, w245, w242, w240) -> (w279:dynamicdata)
        n138 = local write "Voltage Output"(w240) -> ()
        n139 = Merge Signals(w248, w247, w246, w245, w255, w242, w240) -> (w241:dynamicdata)
        n140 = Multiply(x=w271, y=w248) -> (x*y=w268:dynamicdata)
        n141 = Multiply(x=w271, y=w247) -> (x*y=w265:dynamicdata)
        n142 = Multiply(x=w271, y=w246) -> (x*y=w264:dynamicdata)
        n143 = Multiply(x=200.0, y=w245) -> (x*y=w262:dynamicdata)
        n144 = case shown="\"Cold Flow Rig\"" w244 {
          tunnel: w285 -> [w305 w317]
          tunnel: w279 -> [_ w316]
          tunnel: w241 -> [w299 _]
          frame "Test Firing", Default {
            n145 = Build Array("Supply Pressure", "Second Pressure Transducer", "Chamber Pressure", "Volumetric Flow", "Thrust", "Temperature", "Voltage Out" ("element")) -> (w297:string[])
            n146 = call "RenameDynamicSignals.vi"("New Signal Names"=w297, "Dynamic Data In"=w299) -> ("error out"=w295:errorcluster, "Dynamic Data Out"=w296:dynamicdata)  [unwired: 2 in]
            n147 = call "Write To Measurement File3"("Signals"=w296, "Enable"="Collect Data?", "error in (no error)"=w295, "Filename"=w305) -> ("Filename Out"=→"Filename Out":path, "Saving Data"=→"Saving Data":bool, "error out"=→"error out 3":errorcluster)  [unwired: 13 in]
          }
          frame "Cold Flow Rig" {
            n148 = Build Array("Supply Pressure", "Second Pressure Transducer", "Volumetric Flow", "Temperature", "Voltage Out" ("element")) -> (w310:string[])
            n149 = call "RenameDynamicSignals.vi"("New Signal Names"=w310, "Dynamic Data In"=w316) -> ("error out"=w308:errorcluster, "Dynamic Data Out"=w309:dynamicdata)  [unwired: 2 in]
            n150 = call "Write To Measurement File4"("Signals"=w309, "Enable"="Collect Data? 2", "error in (no error)"=w308, "Filename"=w317) -> ("Filename Out"=→"Filename Out":path, "Saving Data"=→"Saving Data":bool)  [unwired: 13 in, 1 out]
          }
        }
        n151 = local write "Supply Pressure PSI"(w268) -> ()
        n152 = local write "Chamber Pressure"(w264) -> ()
        n153 = local write "Second Pressure Transducer"(w265) -> ()
        n154 = local write "Mass Flow L/min"(w262) -> ()
        n155 = call "Convert from Dynamic Data11"("Dynamic Data Type"=w265) -> ("Array"=w266:dbl[])  [unwired: 3 in]
        n156 = call "Convert from Dynamic Data8"("Dynamic Data Type"=w268) -> ("Array"=w267:dbl[])  [unwired: 3 in]
        n157 = call "Convert from Dynamic Data12"("Dynamic Data Type"=w264) -> ("Array"=w263:dbl[])  [unwired: 3 in]
        n158 = call "Convert from Dynamic Data13"("Dynamic Data Type"=w262) -> ("Array"=w261:dbl[])  [unwired: 3 in]
        n159 = call "Convert from Dynamic Data6"() -> ("Array"=w280:dbl[])  [unwired: 4 in]
        n160 = call-poly <vilib>:"Mean.vi"("X"=w280) -> ()  [unwired: 2 out]
        n161 = call-poly <vilib>:"Mean.vi"("X"=w267) -> ("mean"=w260:dbl)  [unwired: 1 out]
        n162 = call-poly <vilib>:"Mean.vi"("X"=w266) -> ("mean"=w259:dbl)  [unwired: 1 out]
        n163 = call-poly <vilib>:"Mean.vi"("X"=w263) -> ("mean"=w258:dbl)  [unwired: 1 out]
        n164 = call-poly <vilib>:"Mean.vi"("X"=w261) -> ("mean"=w257:dbl)  [unwired: 1 out]
        n165 = call "Convert from Dynamic Data3"("Dynamic Data Type"=w242) -> ("Array"=w253:dbl[])  [unwired: 3 in]
        n166 = call "Convert from Dynamic Data4"("Dynamic Data Type"=w240) -> ("Array"=w252:dbl[])  [unwired: 3 in]
        n167 = call "Convert from Dynamic Data"("Dynamic Data Type"=w255) -> ("Array"=w254:dbl[])  [unwired: 3 in]
        n168 = call-poly <vilib>:"Mean.vi"("X"=w252) -> ("mean"=w251:dbl)  [unwired: 1 out]
        n169 = call-poly <vilib>:"Mean.vi"("X"=w254) -> ("mean"=w290:dbl)  [unwired: 1 out]
        n170 = call-poly <vilib>:"Mean.vi"("X"=w253) -> ("mean"=w256:dbl)  [unwired: 1 out]
        n171 = call "Elapsed Time"() -> ("Elapsed Time (s)"=w250:dbl)  [unwired: 12 in, 7 out]
        "Elapsed Time (s)" <- w250
        "Numeric 2" <- w291
      }
      n172 = call <vilib>:"DAQmx Clear Task.vi"("task in"=w53, "error in"=w52) -> ("error out"=→"error out 2":errorcluster)  [unwired: 13 in]
      n173 = Bundle(w32, w31) -> (w30:cluster{dbl[], dbl[]})  [unwired: 1 in]
      "Second Pressure Transducer" <- w30
      n174 = Bundle(w32, w33) -> (w29:cluster{dbl[], dbl[]})  [unwired: 1 in]
      "Chamber Pressure" <- w29
      n175 = Bundle(w32, w40) -> (w38:cluster{dbl[], dbl[]})  [unwired: 1 in]
      "Supply Pressure" <- w38
      n176 = Bundle(w32, w41) -> (w28:cluster{dbl[], dbl[]})  [unwired: 1 in]
      "MassFlow" <- w28
      n177 = Bundle(w32, w39) -> (w27:cluster{dbl[], dbl[]})  [unwired: 1 in]
      "Thrust" <- w27
      n178 = Bundle(w32, w42) -> (w26:cluster{dbl[], dbl[]})  [unwired: 1 in]
      "Temperature" <- w26
      n179 = Bundle(w32, w24) -> (→"Servo Voltage Output":cluster{dbl[], dbl[]})  [unwired: 1 in]
      n180 = Build Array(w38, w30, w29, w28, w27, w26) -> (→"All Channel Graph":cluster{dbl[], dbl[]}[])
    }
  }
